vi "Read PersonnelType.vi"(8 "error in (no error)":errorcluster, 11 "Request in":refnum<class "Request.lvclass">) -> (0 "error out":errorcluster, 2 "PersonnelType":T1 items=["Nurse", "Doctor", "Cleanning", "Admin"], 3 "Request out":refnum<class "Request.lvclass">)   [LabVIEW 2015, in "Request.lvclass"]
uses:
  Request.lvclass
  PersonnelType.ctl
  Request.lvclass/Request.ctl
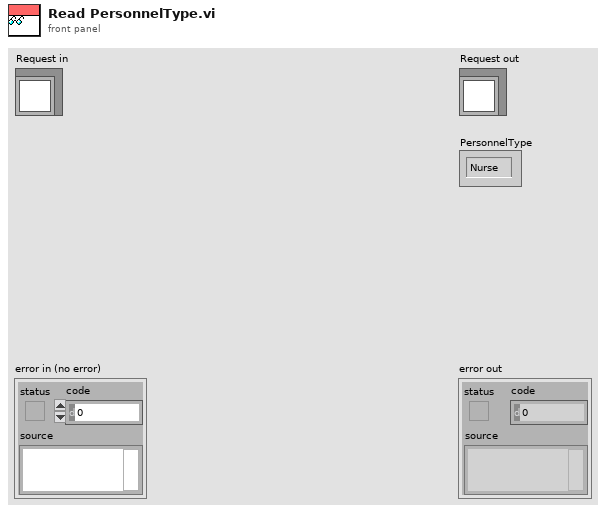
[diagram p1: front panel]
types:
  T1 = typedef "Request.lvclass/PersonnelType.ctl" = u16
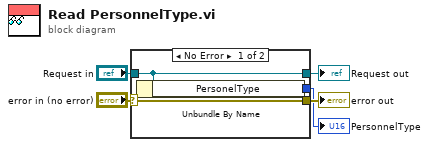
[diagram p0: block diagram]
diagram:
  n1 = case shown="No Error" "error in (no error)" {
    selector: "error in (no error)" -> [w8 w9]
    tunnel: [w8 w9] -> w4
    tunnel: [w7 w10] -> w2
    tunnel: "Request in" -> [w7 w10]
    tunnel: [w6 _] -> w1
    frame No Error {
      n2 = Unbundle By Name(w7) -> ("PersonelType"=w6:T1)
    }
    frame Error {
    }
  }
  "error out" <- w4
  "Request out" <- w2
  "PersonnelType" <- w1
